vi "RichToFlatnixnet_grpc_ReadStateTimeTriggerRequest.vi"(5 "OutputClusterType":T1, 11 "InputCluster":T4) -> (3 "OutputCluster":T1)   [LabVIEW 2025, in "grpc-xnet_client.lvlib"]
uses:
  grpc-xnet_client.lvlib
  nixnet_grpc_ReadStateTimeTriggerRequest.ctl
  nixnet_grpc_ReadStateTimeTriggerRequest_timeout_enum/nixnet_grpc_ReadStateTimeTriggerRequest_timeout_enum.lvclass
  nidevice_grpc_Session.ctl
  nixnet_grpc_ReadStateTimeTriggerRequest_Flat.ctl
  nidevice_grpc_Session_Flat.ctl
  nixnet_grpc_TimeOut.ctl
  nixnet_grpc_ReadStateTimeTriggerRequest_timeout_enum/nixnet_grpc_ReadStateTimeTriggerRequest_timeout_enum.lvclass/nixnet_grpc_ReadStateTimeTriggerRequest_timeout_enum.ctl
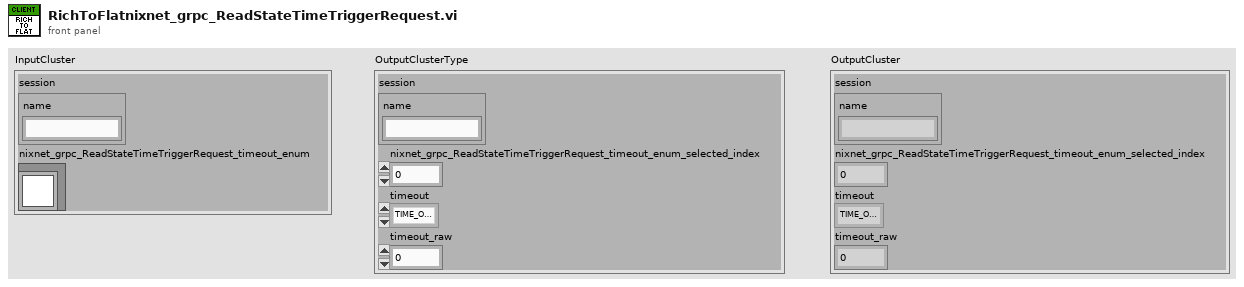
[diagram p1: front panel]
types:
  T1 = typedef "grpc-xnet_client.lvlib/nixnet_grpc_ReadStateTimeTriggerRequest_Flat.ctl" = cluster{"session":T2, "nixnet_grpc_ReadStateTimeTriggerRequest_timeout_enum_selected_index":i32, "timeout":T3, "timeout_raw":dbl}
  T2 = typedef "grpc-xnet_client.lvlib/nidevice_grpc_Session_Flat.ctl" = cluster{"name":string}
  T3 = typedef "grpc-xnet_client.lvlib/nixnet_grpc_TimeOut.ctl" = enum32{"TIME_OUT_NONE", "TIME_OUT_INFINITE"}
  T4 = typedef "grpc-xnet_client.lvlib/nixnet_grpc_ReadStateTimeTriggerRequest.ctl" = cluster{"session":T5, "nixnet_grpc_ReadStateTimeTriggerRequest_timeout_enum":refnum<class "nixnet_grpc_ReadStateTimeTriggerRequest_timeout_enum.lvclass">}
  T5 = typedef "grpc-xnet_client.lvlib/nidevice_grpc_Session.ctl" = cluster{"name":string}
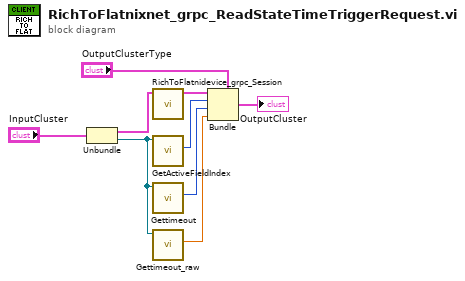
[diagram p0: block diagram]
diagram:
  n1 = Unbundle "Unbundle"("InputCluster") -> ("session"=w6:T5, "nixnet_grpc_ReadStateTimeTriggerRequest_timeout_enum"=w4:refnum<class "nixnet_grpc_ReadStateTimeTriggerRequest_timeout_enum.lvclass">)
  n2 = call "RichToFlatnidevice_grpc_Session.vi"("InputCluster"=w6) -> ("OutputCluster"=w5:T2)  [unwired: 10 in]
  n3 = call "GetActiveFieldIndex.vi"("OneOfTemplate in"=w4) -> ("Active Field Index"=w3:i32)  [unwired: 8 in, 2 out]
  n4 = call "Gettimeout.vi"("OneOfTemplate in"=w4) -> ("Get_Val"=w2:T3)  [unwired: 8 in, 2 out]
  n5 = call "Gettimeout_raw.vi"("OneOfTemplate in"=w4) -> ("Get_Val"=w1:dbl)  [unwired: 8 in, 2 out]
  n6 = Bundle "Bundle"(cluster="OutputClusterType", "session"=w5, "nixnet_grpc_ReadStateTimeTriggerRequest_timeout_enum_selected_index"=w3, "timeout"=w2, "timeout_raw"=w1) -> (→"OutputCluster":T1)
